vi "624WPI Dashboard Video Path.vi"(11 "Camera IP":string) -> (3 "Video Path":path)   [LabVIEW 2013]
uses:
  <vilib>/Rock Robotics/WPI/Dashboard/WPI_DashboardLogging Global.vi
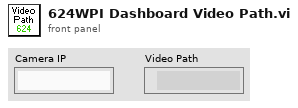
[diagram p1: front panel]
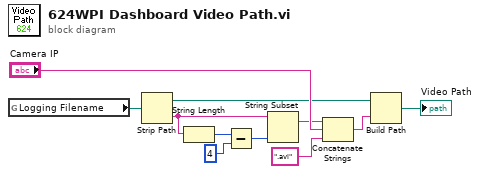
[diagram p0: block diagram]
diagram:
  n1 = global read "WPI_DashboardLogging Global.vi" "Logging Filename"() -> (w2:path)
  n2 = Strip Path(path=w2) -> (stripped path=w3:path, name=w11:string)
  n3 = String Length(string=w11) -> (length=w4:i32)
  n4 = Subtract(x=w4, y=4) -> (x-y=w6:i32)
  n5 = String Subset(string=w11, length (rest)=w6) -> (substring=w8:string)  [unwired: 1 in]
  n6 = Concatenate Strings(w8, "Camera IP", ".avi") -> (w10:string)
  n7 = Build Path(base path=w3, name or relative path=w10) -> (appended path=→"Video Path":path)
